vi "Energy_GUI.vi"(10 "stop 2":refnum<vi>, 11 "GUI_cluster":T3={"Sub Panel"=refnum, "GUIdevice"="Bella_LP_Mode", "CtlRef"=refnum, "user event out"=refnum}) -> ()   [LabVIEW 2011]
uses:
  GUI_Template/GUI_master/tcp_new_data_event.ctl
  GUI_Template/GUI_master/tcp new data cluster.ctl
  Controls/GUI_cluster.ctl
  Controls/eventtypdef.ctl
  Device Driver/StagingAnalysis/SubVis/SubVi/polTypDef.ctl
  Device Driver/shared/OnOffTypeDef.ctl
  Device Driver/StagingAnalysis/SubVis/energyCalibTypdef.ctl
  <vilib>/Analysis/1siggen.llb/Ramp Pattern by Samples.vi
  Device Driver/BaseDriver/BaseDriver.lvclass
  <vilib>/Analysis/NI_AALBase.lvlib
panel:
  in  "Beamselectr":u16(ring) items=["Beam1", "Beam2"]
  in  "tapsselector":u16(ring) items=["Transmission", "Raw Data"]
  in  "Tab Control":enum32{"Transmission", "raw"}(tab)
  out "Chart":dbl(graph) caption="Transmission Beam1"
  out "XY Graph":cluster{"Ramp Pattern":dbl[], "f(X, a)":dbl[]}[](graph)
  in  "plotb calib":bool
  in  "ok::1":T1
  out "Polarization::1":T2
  out "BCaveFilterStatus::1":enum16{"B-Cave filter in", "B-Cave filter out"}(ring)
  in  "EnergyIn::1":dbl caption="Energy in (raw)" min=0.0 max=0.0 format="%#_6p"
  in  "Energy out (raw)::1":dbl caption="Energy out (raw)" min=0.0 max=0.0 format="%#_6p"
  in  "EnergyOut::1":dbl caption="EnergyOut (mJ)" min=0.0 max=0.0 format="%#_6p"
  in  "EnergyTransmission Beam 2::1":dbl caption="Beam 2" min=0.0 max=0.0
  in  "EnergyTransmission Beam 1::1":dbl caption="Beam1" min=0.0 max=0.0
  out "tcp data event":T4
  out "GUIdevice 1":string="Bella_LP_Mode"
  in  "stop":bool
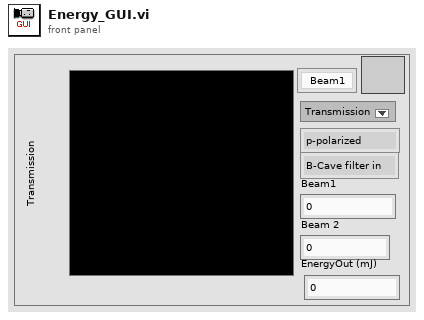
[diagram p1: front panel]
types:
  T1 = typedef "OnOffTypeDef.ctl" = enum16{"off", "on"}
  T2 = typedef "polTypDef.ctl" = enum16{"p-polarized", "s-polarized"}
  T3 = typedef "GUI_cluster.ctl" = cluster{"Sub Panel":refnum<vi>, "GUIdevice":string, "CtlRef":refnum<vi>, "user event out":refnum<user-event>}
  T4 = typedef "tcp_new_data_event.ctl" = refnum<user-event>
  T5 = typedef "energyCalibTypdef.ctl" = cluster{"p-pol":cluster{"Beam1":dbl, "Beam2":dbl, "Tele":dbl, "startLinear":dbl, "best fit parameters":cluster{"0":dbl, "1":dbl, "2":dbl, "3":dbl}}, "s-pol":cluster{"Beam1":dbl, "Beam2":dbl, "Tele":dbl, "position for fit":dbl, "best fit parameters":cluster{"0":dbl, "1":dbl, "2":dbl, "3":dbl}}, "B-CaveFilter":dbl}
  T6 = typedef "eventtypdef.ctl" = cluster{"label":string, "Sub Panel":refnum<vi>, "CtlRef":refnum<vi>, "This VI":refnum<vi>}
  T7 = typedef "tcp new data cluster.ctl" = cluster{"EventEnum":enum16{"new data", "connection status update"}, "Device name":string}
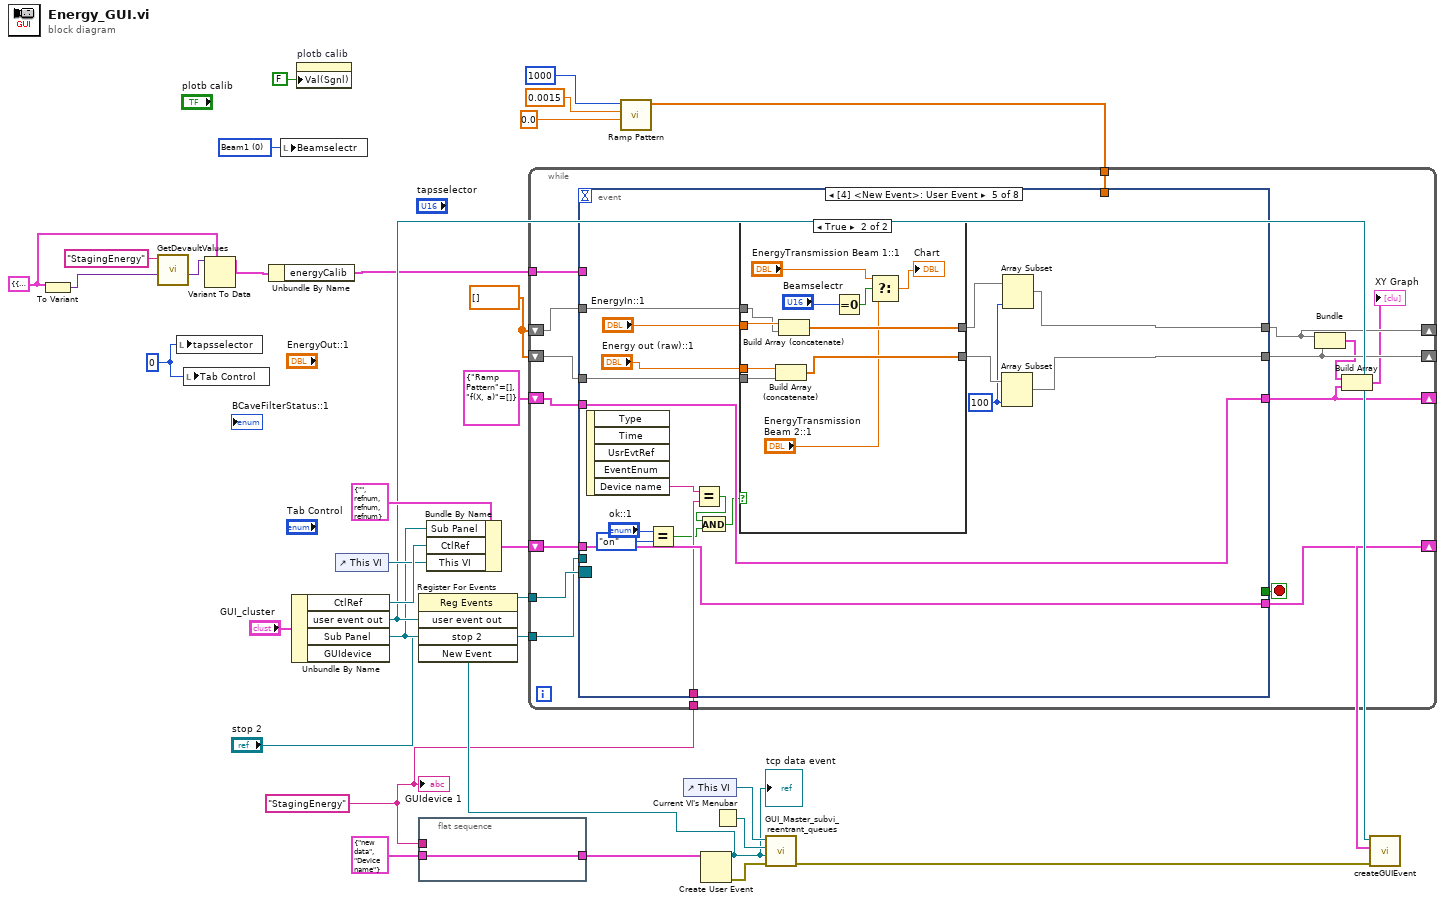
[diagram p0: block diagram]
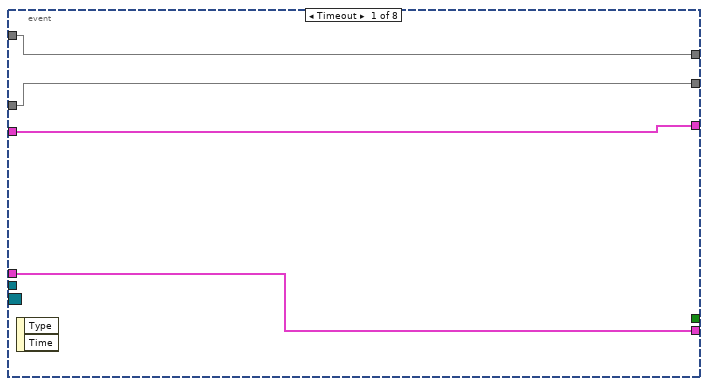
[diagram p2: hidden frame]
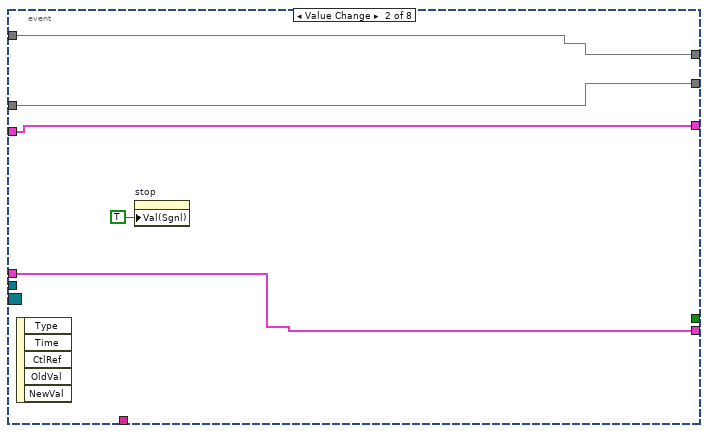
[diagram p3: hidden frame]
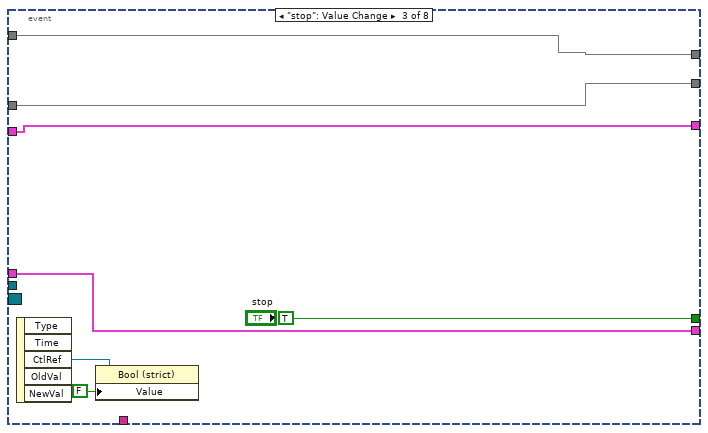
[diagram p4: hidden frame]
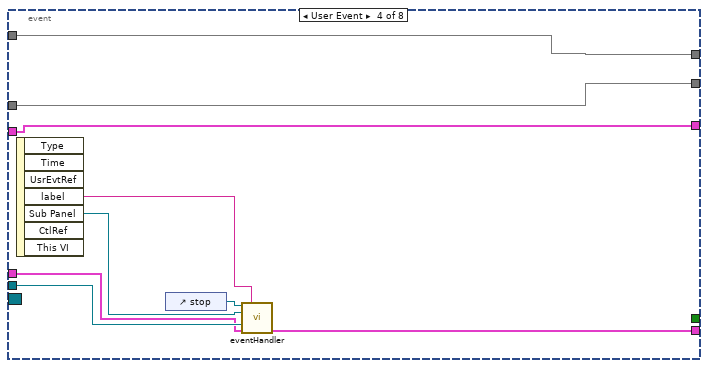
[diagram p5: hidden frame]
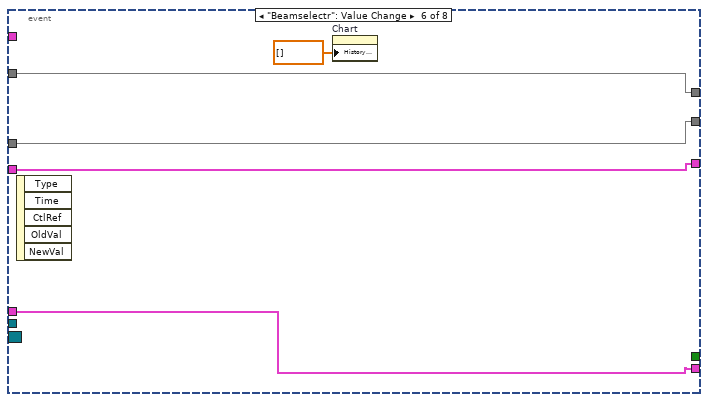
[diagram p7: hidden frame]
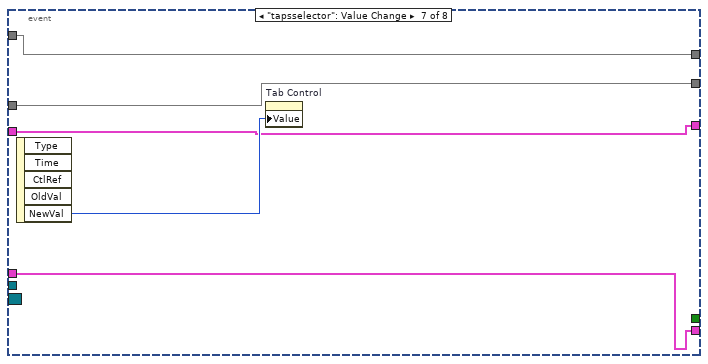
[diagram p8: hidden frame]
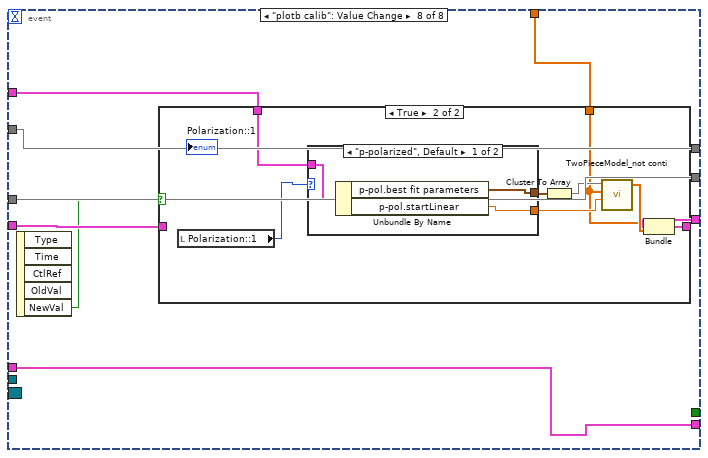
[diagram p9: hidden frame]
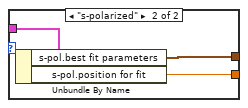
[diagram p11: hidden frame]
diagram:
  w1 = u16 0 items=["Beam1", "Beam2"] ("Beamselectr")
  w2 = 0
  w13 = cluster{"energyCalib":T5} {"energyCalib"={"p-pol"={"Beam1"=0.24495733496510103, "Beam2"=0.755042665034899, "Tele"=0.06901139685565201, "startLinear"=0.0007, "best fit parameters"={"0"=0.06577078607141854, "1"=1075.8816653301244, "2"=-1751262.2505806182, "3"=1069290462.0527091}}, "s-pol"={"Beam1"=0.5855752916708905, "Beam2"=0.4144247083291095, "Tele"=0.004937888283292143, "position for fit"=0.0007, "best fit parameters"={"0"=0.024167, "1"=188.618, "2"=-273128.0, "3"=156332000.0}}, "B-CaveFilter"=0.89}}
  w15 = dbl[] []
  w16 = "StagingEnergy"
  n1 = To Variant(anything=w13) -> (Variant=w10:variant)
  n2 = call "GetDevaultValues.vi"("variant"=w10, "Device Name"="StagingEnergy") -> ("variant out"=w11:variant)  [unwired: 7 in, 2 out]
  n3 = local write "tapsselector"(w2) -> ()
  n4 = local write "Tab Control"(w2) -> ()
  n5 = Variant To Data(type=w13, Variant=w11) -> (data=w12:cluster{"energyCalib":T5})  [unwired: 1 in, 1 out]
  n6 = Unbundle By Name(w12) -> ("energyCalib"=w9:T5)
  n7 = local write "Beamselectr"(w1) -> ()
  n8 = Unbundle By Name("GUI_cluster") -> ("CtlRef"=w26:refnum<vi>, "user event out"=w22:refnum<user-event>, "Sub Panel"=w20:refnum<vi>)  [unwired: 1 out]
  n9 = property on="plotb calib" class="Bool (strict)"("Val(Sgnl)"=FALSE ("Value (Signaling)")) -> ()  [unwired: 2 in, 2 out]
  n10 = control-ref of="This VI"() -> (w25:refnum<vi>)
  n11 = flat-sequence {
    tunnel: T7 {"EventEnum"=enum."new data", "Device name"="Device name"} ("New Event") -> [w34]
    tunnel: [w34] -> w27
    tunnel: w16 -> [_]
    frame #0 {
    }
  }
  n12 = Bundle By Name(cluster=T6 {"label"="", "Sub Panel"=refnum, "CtlRef"=refnum, "This VI"=refnum} ("event data"), "Sub Panel"=w20, "CtlRef"=w26, "This VI"=w25) -> (w23:T6)
  n13 = call-poly <vilib>:"Ramp Pattern.vi"("start"=0.0, "end"=0.0015, "samples"=1000) -> ("Ramp Pattern"=w5:dbl[])  [unwired: 7 in, 1 out]
  n14 = control-ref of="This VI"() -> (w33:refnum<vi>)
  n15 = Create User Event(user event datatype=w27) -> (user event=w17:refnum<user-event>, error out=w31:errorcluster)  [unwired: 1 in]
  "tcp data event" <- w17
  n16 = register-events(w22, "stop 2", w17) -> (reference out=w21:refnum<event-registration>)  [unwired: 2 in, 1 out]
  n17 = while {
    shift-right: [w48] -> w19
    shift-left: w23 -> [w49]
    tunnel: w21 -> [w47]
    tunnel: w20 -> [w46]
    tunnel: w16 -> [w45]
    shift-right: [w42] -> _
    shift-left: w15 -> [w44]
    shift-right: [w41] -> _
    shift-left: w15 -> [w43]
    tunnel: w9 -> [w40]
    tunnel: w5 -> [w39]
    shift-right: [w36] -> _
    shift-left: cluster{"Ramp Pattern":dbl[], "f(X, a)":dbl[]} {"Ramp Pattern"=[], "f(X, a)"=[]} -> [w38]
    stop <- w50 stop-if-true
    n18 = event shown="[4] <New Event>: User Event" {
      selector: w47 -> [_ _ _ _ _ _ _ _]
      dyn-events: _ -> [_ _ _ _ _ _ _ _]
      timeout: _ -> [_ _ _ _ _ _ _ _]
      tunnel: [_ _ TRUE ("stop") _ _ _ _ _] -> w50
      tunnel: w49 -> [w54 w59 w66 w72 w93 w108 w113 w122]
      tunnel: [w54 w59 w66 w71 w93 w108 w113 w122] -> w48
      tunnel: w46 -> [_ _ _ w73 _ _ _ _]
      tunnel: w45 -> [_ _ _ _ w91 _ _ _]
      tunnel: [w53 w57 w62 w69 w82 w111 w115 w124] -> w42
      tunnel: w44 -> [w53 w57 w62 w69 w89 w111 w115 w124]
      tunnel: w43 -> [w52 w56 w61 w68 w87 w110 w114 w123]
      tunnel: [w52 w56 w61 w68 w83 w110 w114 w123] -> w41
      tunnel: w40 -> [_ _ _ _ _ _ _ w121]
      tunnel: w39 -> [_ _ _ _ _ _ _ w120]
      tunnel: [w51 w55 w60 w67 w81 w109 w112 w119] -> w36
      tunnel: w38 -> [w51 w55 w60 w67 w81 w109 w112 w118]
      event Timeout {
        n19 = event-data() -> ()  [unwired: 1 in, 2 out]
      }
      event Value Change {
        n20 = event-data() -> ()  [unwired: 1 in, 5 out]
        n21 = property on="stop" class="Bool (strict)"("Val(Sgnl)"=TRUE ("Value (Signaling)")) -> ()  [unwired: 2 in, 2 out]
      }
      event "stop": Value Change {
        n22 = event-data() -> ("CtlRef"=w65:refnum<vi>)  [unwired: 1 in, 4 out]
        n23 = property class="Bool (strict)"(reference=w65, "Value"=FALSE) -> ()  [unwired: 1 in, 2 out]
      }
      event User Event {
        n24 = event-data() -> ("label"=w70:string, "Sub Panel"=w74:refnum<vi>)  [unwired: 1 in, 5 out]
        n25 = control-ref of="stop"() -> (w75:refnum<vi>)
        n26 = call "eventHandler.vi"("Boolean in"=w75, "label"=w70, "Sub Panel 2"=w74, "Sub Panel"=w73, "event data in"=w72) -> ("event data out"=w71:T6)  [unwired: 10 in]
      }
      event User Event {
        w84 = 100 ("length")
        n27 = event-data() -> ("Device name"=w92:string)  [unwired: 1 in, 4 out]
        n28 = Equal?(x="ok::1", y=OnOffTypeDef."on") -> (x = y?=w77:bool)
        n29 = Equal?(x=w92, y=w91) -> (x = y?=w78:bool)
        n30 = And(x=w78, y=w77) -> (x .and. y?=w76:bool)
        n31 = case shown="True" w76 {
          tunnel: "EnergyIn::1" -> [_ w104]
          tunnel: [w95 w106] -> w86
          tunnel: w89 -> [w95 w103]
          tunnel: "Energy out (raw)::1" -> [_ w102]
          tunnel: w87 -> [w94 w101]
          tunnel: [w94 w105] -> w85
          frame False {
          }
          frame True {
            n32 = Build Array (concatenate)(w102, w101) -> (w105:dbl[])
            n33 = Build Array (concatenate)(w104, w103) -> (w106:dbl[])
            n34 = Equal To 0?(x="Beamselectr") -> (x = 0?=w99:bool)
            n35 = Select(t="EnergyTransmission Beam 1::1", s=w99, f="EnergyTransmission Beam 2::1") -> (s? t:f=→"Chart":dbl)
          }
        }
        n36 = Array Subset(array=w85, length=w84) -> (w83:dbl[])  [unwired: 1 in]
        n37 = Array Subset(array=w86, length=w84) -> (w82:dbl[])  [unwired: 1 in]
      }
      event "Beamselectr": Value Change {
        n38 = event-data() -> ()  [unwired: 1 in, 5 out]
        n39 = property on="Chart" class="WFChart (strict)"("History Data"=dbl[] []) -> ()  [unwired: 2 in, 2 out]
      }
      event "tapsselector": Value Change {
        n40 = event-data() -> ("NewVal"=w116:u16)  [unwired: 1 in, 4 out]
        n41 = property on="Tab Control" class="TabCtl (strict)"("Value"=w116) -> ()  [unwired: 2 in, 2 out]
      }
      event "plotb calib": Value Change {
        n42 = event-data() -> ("NewVal"=w117:bool)  [unwired: 1 in, 4 out]
        n43 = case shown="True" w117 {
          tunnel: w121 -> [_ w133]
          tunnel: [w125 w128] -> w119
          tunnel: w120 -> [_ w127]
          tunnel: w118 -> [w125 _]
          frame False {
          }
          frame True {
            n44 = local read "Polarization::1"() -> (w126:T2)
            n45 = case shown="\"p-polarized\", Default" w126 {
              tunnel: w133 -> [w136 w139]
              tunnel: [w135 w138] -> w132
              tunnel: [w134 w137] -> w130
              frame "p-polarized", Default {
                n46 = Unbundle By Name(w136) -> ("p-pol.best fit parameters"=w135:cluster{"0":dbl, "1":dbl, "2":dbl, "3":dbl}, "p-pol.startLinear"=w134:dbl)
              }
              frame "s-polarized" {
                n47 = Unbundle By Name(w139) -> ("s-pol.best fit parameters"=w138:cluster{"0":dbl, "1":dbl, "2":dbl, "3":dbl}, "s-pol.position for fit"=w137:dbl)
              }
            }
            n48 = Cluster To Array(cluster=w132) -> (array=w131:dbl[])
            n49 = call "TwoPieceModel_not conti.vi"("data"=w130, "x"=w127, "a"=w131) -> ("f(X, a)"=w129:dbl[])  [unwired: 1 in, 2 out]
            n50 = Bundle("Ramp Pattern"=w127, "f(X, a)"=w129) -> (w128:cluster{"Ramp Pattern":dbl[], "f(X, a)":dbl[]})  [unwired: 1 in]
          }
        }
      }
    }
    n51 = Bundle(w42, w41) -> (w37:cluster{dbl[], dbl[]})  [unwired: 1 in]
    n52 = Build Array(w37, w36) -> (→"XY Graph":cluster{"Ramp Pattern":dbl[], "f(X, a)":dbl[]}[])
  }
  n53 = Current VI's Menubar() -> (w32:refnum<k9>)
  n54 = call "GUI_Master_subvi_reentrant_queues.vi"("error in (no error)"=w31, "tcp data event"=w17, "Caller menu reference"=w32, "Caller VI ref"=w33) -> ("error out"=w24:errorcluster)  [unwired: 7 in]
  n55 = call "createGUIEvent.vi"("error in (no error)"=w24, "event data"=w19, "User Event in"=w22) -> ()  [unwired: 9 in]
  "GUIdevice 1" <- w16
